vi "P4CMD Dialog - Submit.vi"(6 "changelist files":string[](array[string]), 7 "operation info":T1, 8 "error in (no error)":errorcluster, 9 "description in":string, 10 "input files":string[](array[string])) -> (0 "error out":errorcluster, 1 "description out":string, 2 "filtered file list":string[](array[string]), 5 "dialog box cancelled?":bool)   [LabVIEW 2017, in "NI_SCC_P4CMD.lvlib"]
uses:
  <vilib>/SourceControl/Providers/P4CMD/NI_SCC_P4CMD.lvlib
  <vilib>/SourceControl/support/SCCSup Message Strings GLBL.vi
panel:
  out "submit msg":string="Submit open files to the depot"
  out "Changelist:":string
  out "Date:":string
  out "Client:":string
  out "User:":string
  out "Status:":string
  in  "Description:":string="<enter description here>"
  in  "Cancel":bool
  in  "OK":bool
  in  "Help":bool
  in  "CheckNone":bool
  in  "CheckAll":bool
  in  "Files:":i32[](listbox)
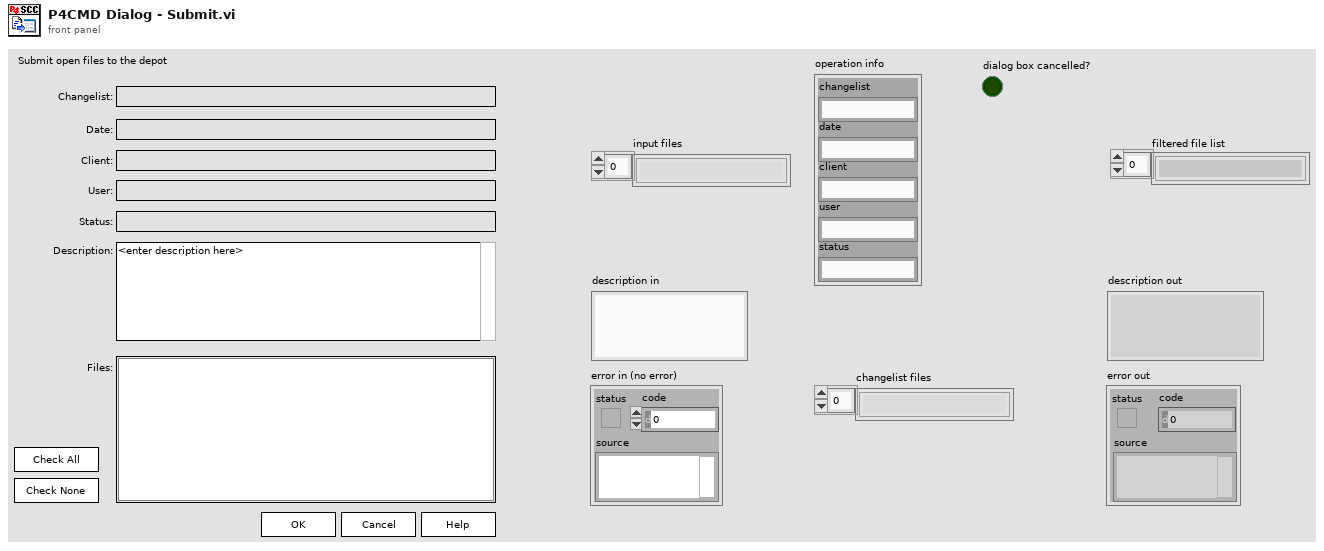
[diagram p1: front panel]
types:
  T1 = cluster{"changelist":string, "date":string, "client":string, "user":string, "status":string}
  T2 = enum16{"Get Checked Symbol", "Get Unchecked Symbol", "Toggle Symbol"}
  T3 = cluster{"Left Button Key Shortcut":cluster{"Control":bool, "Shift":bool, "Key":string}, "Center Button Key Shortcut":cluster{"Control":bool, "Shift":bool, "Key":string}, "Right Button Key Shortcut":cluster{"Control":bool, "Shift":bool, "Key":string}}
  T4 = enum32{"Invalid", "Standard", "Closed", "Hidden", "Minimized", "Maximized"}
  T5 = typedef "LVPoint32TypeDef.ctl" = cluster{"Horizontal":i32, "Vertical":i32}
  T6 = enum16{"Left Button", "Center Button", "Right Button", "Window Close"}
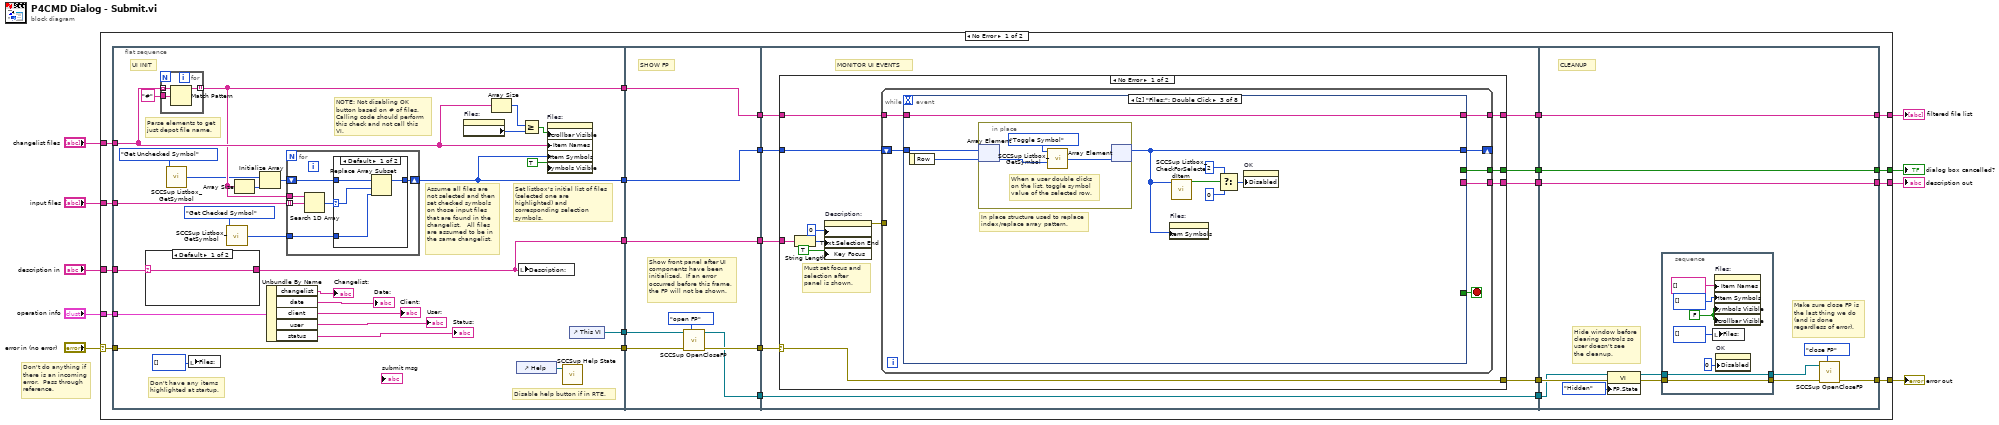
[diagram p0: block diagram]
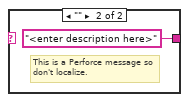
[diagram p2: hidden frame]
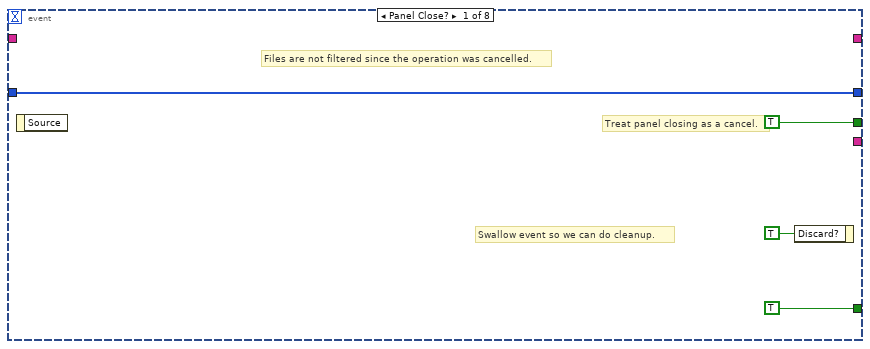
[diagram p4: hidden frame]
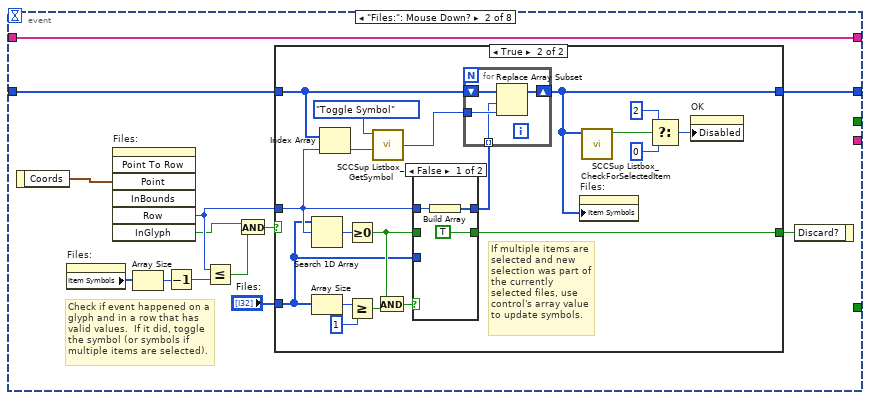
[diagram p5: hidden frame]
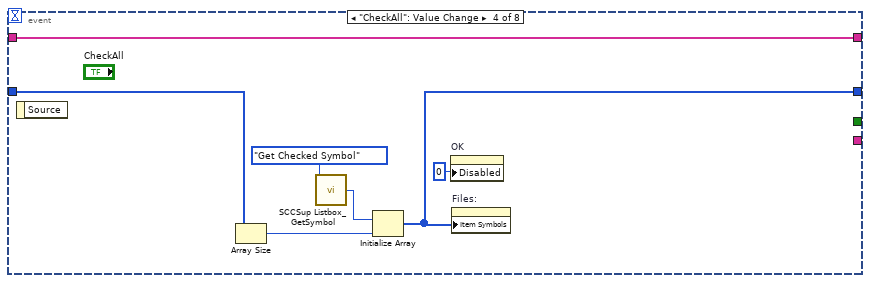
[diagram p8: hidden frame]
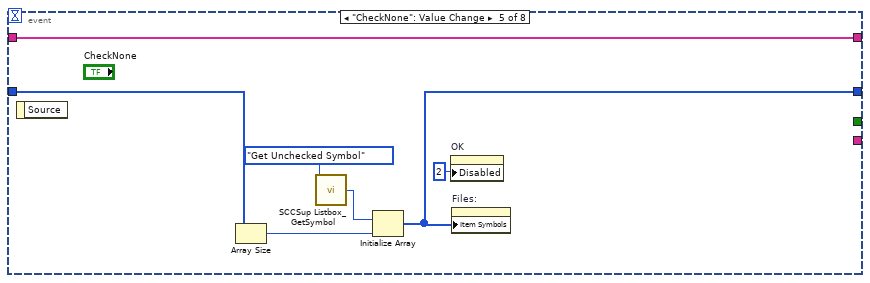
[diagram p9: hidden frame]
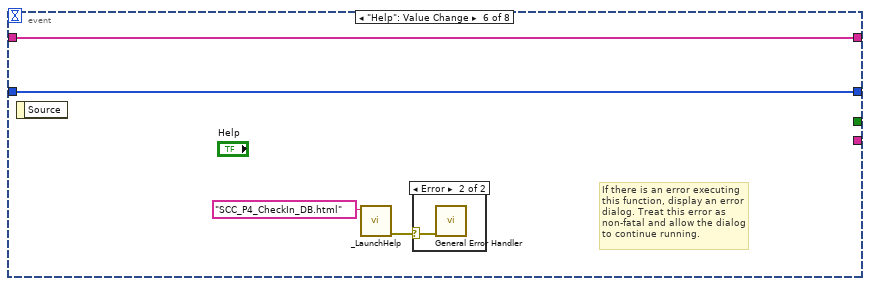
[diagram p10: hidden frame]
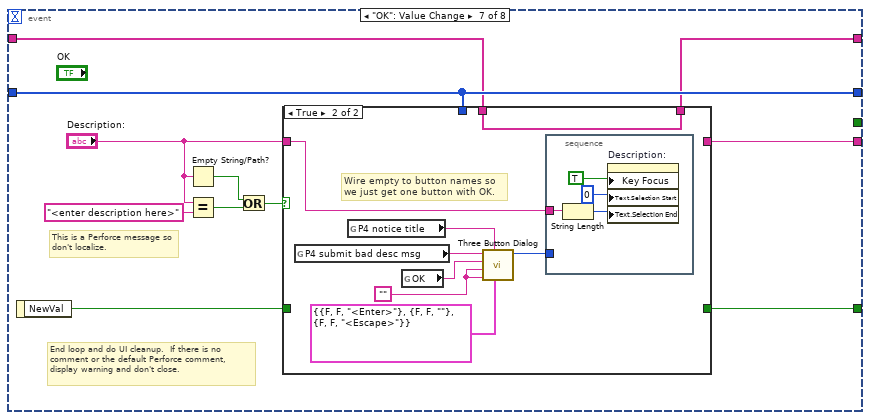
[diagram p12: hidden frame]
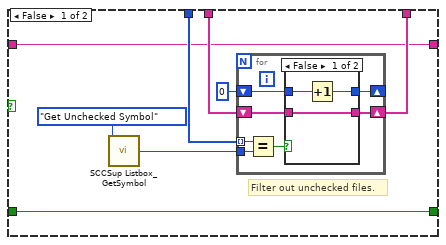
[diagram p13: hidden frame]
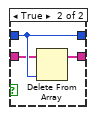
[diagram p14: hidden frame]
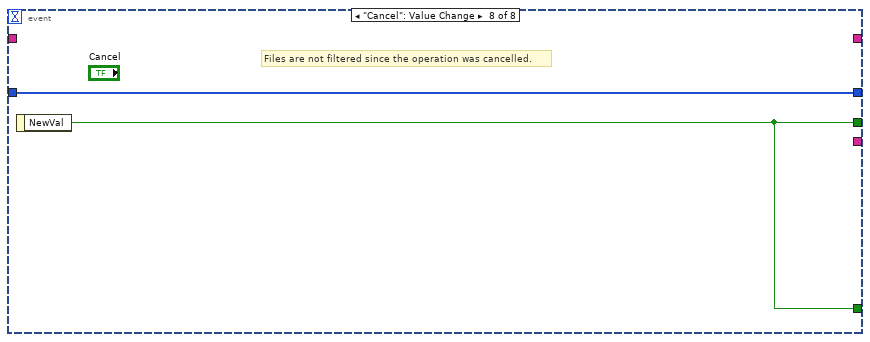
[diagram p15: hidden frame]
diagram:
  # "Don't do anything if there is an incoming error.  Pass through reference."
  n1 = case shown="No Error" "error in (no error)" {
    selector: "error in (no error)" -> [w20 w254]
    tunnel: [w24 w254] -> w9
    tunnel: [w23 _] -> w1
    tunnel: [w22 _] -> w8
    tunnel: [w21 _] -> w7
    tunnel: "input files" -> [w17 _]
    tunnel: "operation info" -> [w16 _]
    tunnel: "description in" -> [w15 _]
    tunnel: "changelist files" -> [w14 _]
    frame No Error {
      n2 = flat-sequence {
        tunnel: [w38] -> w33
        tunnel: [w40] -> w32
        tunnel: [w37] -> w31
        tunnel: w20 -> [w38]
        tunnel: [w47] -> w19
        tunnel: w17 -> [w46]
        tunnel: w16 -> [w57]
        tunnel: w15 -> [w39]
        tunnel: w14 -> [w51]
        tunnel: [w34] -> w11
        tunnel: w33 -> [w82]
        tunnel: w32 -> [w84]
        tunnel: [w84] -> w30
        tunnel: [w83] -> w29
        tunnel: w31 -> [w81]
        tunnel: w19 -> [w83]
        tunnel: [w79] -> w18
        tunnel: [w78] -> w13
        tunnel: w11 -> [w77]
        tunnel: [w77] -> w10
        tunnel: w30 -> [w92]
        tunnel: w29 -> [w93]
        tunnel: [w87] -> w28
        tunnel: [w91] -> w27
        tunnel: [w90] -> w26
        tunnel: [w89] -> w25
        tunnel: w18 -> [w88]
        tunnel: w13 -> [w86]
        tunnel: [w86] -> w12
        tunnel: w10 -> [w85]
        tunnel: [w235] -> w24
        tunnel: w28 -> [w246]
        tunnel: [w244] -> w23
        tunnel: w27 -> [w244]
        tunnel: w26 -> [w243]
        tunnel: [w243] -> w22
        tunnel: w25 -> [w242]
        tunnel: [w242] -> w21
        tunnel: w12 -> [w240]
        frame #0 {
          # "Disable help button if in RTE."
          # "Set listbox's initial list of files (selected one are highlighted) and corresponding selection symbols."
          # "Assume all files are not selected and then set checked symbols on those input files that are found in the changelist.   All files are assumed to be in the same changelist."
          # "Don't have any items highlighted at startup."
          # "Parse elements to get just depot file name."
          # "UI INIT"
          # "NOTE: Not disabling OK button based on # of files.  Calling code should perform this check and not call this VI."
          n3 = case shown="Default" w39 {
            selector: w39 -> [w61 _]
            tunnel: [w61 "<enter description here>" ("Description:")] -> w34
            frame Default {
            }
            frame "" {
              # "This is a Perforce message so don't localize."
            }
          }
          n4 = for {
            tunnel: w51 -> [w76] mode=indexing
            tunnel: [w75] -> w47 mode=indexing
            tunnel: "#" ("regular expression") -> [w74]
            n5 = Match Pattern(string=w76, regular expression=w74) -> (before substring=w75:string)  [unwired: 1 in, 3 out]
          }
          n6 = call <vilib>:"SCCSup Listbox_GetSymbol.vi"("operation"=T2."Get Unchecked Symbol") -> ("symbol out"=w41:i32)  [unwired: 6 in]
          n7 = local write "Files:"(i32[] []) -> ()
          n8 = call <vilib>:"SCCSup Listbox_GetSymbol.vi"("operation"=T2."Get Checked Symbol") -> ("symbol out"=w42:i32)  [unwired: 6 in]
          n9 = Array Size(array=w47) -> (size(s)=w48:i32)
          n10 = Initialize Array(w41, w48) -> (w49:i32[])
          n11 = Unbundle By Name(w57) -> ("changelist"=→"Changelist:":string, "date"=→"Date:":string, "client"=→"Client:":string, "user"=→"User:":string, "status"=→"Status:":string)
          n12 = for {
            tunnel: w47 -> [w68]
            tunnel: w46 -> [w67] mode=indexing
            shift-right: [w64] -> w40
            shift-left: w49 -> [w65]
            tunnel: w42 -> [w63]
            n13 = Search 1D Array(1D array=w68, element=w67) -> (index of element=w66:i32)  [unwired: 1 in]
            n14 = case shown="Default" w66 {
              selector: w66 -> [w70 _]
              tunnel: w65 -> [w72 w73]
              tunnel: [w71 w73] -> w64
              tunnel: w63 -> [w69 _]
              frame Default {
                n15 = Replace Array Subset(array=w72, new element=w69, index=w70) -> (w71:i32[])
              }
              frame -1 {
              }
            }
          }
          n16 = property on="Files:" class="LstBox (strict)"() -> ("Number of Rows"=w36:u32)  [unwired: 2 in, 2 out]
          n17 = Array Size(array=w51) -> (size(s)=w60:i32)
          n18 = control-ref of="Help"() -> (w35:refnum<vi>)
          n19 = local write "Description:"(w34) -> ()
          n20 = Greater Or Equal?(x=w60, y=w36) -> (x >= y?=w58:bool)
          n21 = property on="Files:" class="LstBox (strict)"("Scrollbar Visible"=w58, "Item Names"=w51, "Item Symbols"=w40, "Symbols Visible"=TRUE) -> ()  [unwired: 2 in, 2 out]
          n22 = call <vilib>:"SCCSup Help State.vi"("help ref"=w35) -> ()  [unwired: 10 in, 1 out]
          n23 = control-ref of="This VI"() -> (w37:refnum<vi>)
        }
        frame #1 {
          # "SHOW FP"
          # "Show front panel after UI components have been initialized.  If an error occurred before this frame, the FP will not be shown."
          n24 = call <vilib>:"SCCSup OpenCloseFP.vi"("function"=enum16{"open FP", "close FP"}."open FP", "error in (no error)"=w82, "VI Refnum in"=w81) -> ("error out"=w79:errorcluster, "VI Refnum out"=w78:refnum<vi>)  [unwired: 7 in]
        }
        frame #2 {
          # "MONITOR UI EVENTS"
          n25 = case shown="No Error" w88 {
            selector: w88 -> [w99 w234]
            tunnel: w93 -> [w104 _]
            tunnel: w92 -> [w103 _]
            tunnel: [w102 _] -> w91
            tunnel: [w101 _] -> w90
            tunnel: [w100 _] -> w89
            tunnel: [w99 w234] -> w87
            tunnel: w85 -> [w95 _]
            frame No Error {
              # "Must set focus and selection after panel is shown."
              n26 = String Length(string=w95) -> (length=w98:i32)
              n27 = property on="Description:" class="Str"("Text.Selection Start"=u32 0 ("Text.Selection:Start"), "Text.Selection End"=w98, "Key Focus"=TRUE) -> (error out=w94:errorcluster)  [unwired: 2 in, 1 out]
              n28 = while {
                tunnel: w104 -> [w111]
                shift-right: [w109] -> _
                shift-left: w103 -> [w110]
                tunnel: [w108] -> w102
                tunnel: [w107] -> w101
                tunnel: [w105] -> w100
                tunnel: w94 -> [_]
                stop <- w106 stop-if-true
                n29 = event shown="[2] \"Files:\": Double Click" {
                  selector: _ -> [_ _ _ _ _ _ _ _]
                  dyn-events: _ -> [_ _ _ _ _ _ _ _]
                  timeout: _ -> [_ _ _ _ _ _ _ _]
                  tunnel: w111 -> [_ w125 w165 w175 w182 w186 w197 _]
                  tunnel: w110 -> [w115 w119 w160 w172 w177 w185 w198 w232]
                  tunnel: [w115 w121 w158 w169 w176 w185 w198 w232] -> w109
                  tunnel: [_ w125 w165 w175 w182 w186 w196 _] -> w108
                  tunnel: [TRUE ("Discard?") _ _ _ _ _ _ w233] -> w107
                  tunnel: [TRUE ("Discard?") _ _ _ _ _ w188 w233] -> w106
                  tunnel: [_ _ _ _ _ _ w193 _] -> w105
                  event Panel Close? {
                    # "Treat panel closing as a cancel."
                    # "Files are not filtered since the operation was cancelled."
                    # "Swallow event so we can do cleanup."
                    n30 = event-data() -> ()  [unwired: 1 in, 1 out]
                    n31 = event-data("Discard?"=TRUE) -> ()  [unwired: 1 in, 1 out]
                  }
                  event "Files:": Mouse Down? {
                    # "Check if event happened on a glyph and in a row that has valid values.  If it did, toggle the symbol (or symbols if multiple items are selected)."
                    n32 = event-data() -> ("Coords"=w116:T5)  [unwired: 1 in]
                    n33 = property on="Files:" class="LstBox (strict)"() -> ("Item Symbols"=w128:i32[])  [unwired: 2 in, 2 out]
                    n34 = invoke on="Files:" class="LstBox (strict)" method="Point To Row"("Point"=w116) -> ("Row"=w118:i32, "InGlyph"=w117:bool)  [unwired: 6 in, 5 out]
                    n35 = Array Size(array=w128) -> (size(s)=w120:i32)
                    n36 = Decrement(x=w120) -> (x-1=w127:i32)
                    n37 = Less Or Equal?(x=w118, y=w127) -> (x <= y?=w126:bool)
                    n38 = And(x=w117, y=w126) -> (x .and. y?=w124:bool)
                    n39 = case shown="True" w124 {
                      tunnel: "Files:" -> [_ w139]
                      tunnel: w118 -> [_ w140]
                      tunnel: w119 -> [w129 w137]
                      tunnel: [_ w138] -> w122
                      tunnel: [w129 w134] -> w121
                      frame False {
                      }
                      frame True {
                        # "If multiple items are selected and new selection was part of the currently selected files, use control's array value to update symbols."
                        n40 = Search 1D Array(1D array=w139, element=w140) -> (index of element=w146:i32)  [unwired: 1 in]
                        n41 = Array Size(array=w139) -> (size(s)=w148:i32)
                        n42 = Index Array(array=w137, index=w140) -> (element=w144:i32)
                        n43 = Greater Or Equal To 0?(x=w146) -> (x >= 0?=w141:bool)
                        n44 = Greater Or Equal?(x=w148, y=1) -> (x >= y?=w145:bool)
                        n45 = call <vilib>:"SCCSup Listbox_GetSymbol.vi"("operation"=T2."Toggle Symbol", "symbol in"=w144) -> ("symbol out"=w136:i32)  [unwired: 5 in]
                        n46 = And(x=w141, y=w145) -> (x .and. y?=w142:bool)
                        n47 = case shown="False" w142 {
                          tunnel: w141 -> [_ w156]
                          tunnel: w140 -> [w155 _]
                          tunnel: w139 -> [_ w157]
                          tunnel: [w154 w157] -> w135
                          tunnel: [TRUE w156] -> w138
                          frame False {
                            n48 = Build Array(w155) -> (w154:i32[])
                          }
                          frame True {
                          }
                        }
                        n49 = for {
                          shift-right: [w151] -> w134
                          shift-left: w137 -> [w152]
                          tunnel: w136 -> [w150]
                          tunnel: w135 -> [w149] mode=indexing
                          n50 = Replace Array Subset(array=w152, new element=w150, index=w149) -> (w151:i32[])
                        }
                        n51 = property on="Files:" class="LstBox (strict)"("Item Symbols"=w134) -> ()  [unwired: 2 in, 2 out]
                        n52 = call <vilib>:"SCCSup Listbox_CheckForSelectedItem.vi"("symbols array"=w134) -> ("item selected?"=w131:bool)  [unwired: 9 in, 1 out]
                        n53 = Select(t=u8 2 ("Disabled"), s=w131, f=u8 0) -> (s? t:f=w130:u8)
                        n54 = property on="OK" class="Bool"("Disabled"=w130) -> ()  [unwired: 2 in, 2 out]
                      }
                    }
                    n55 = event-data("Discard?"=w122) -> ()  [unwired: 1 in, 1 out]
                  }
                  event "Files:": Double Click {
                    # "In place structure used to replace index/replace array pattern."
                    n56 = event-data() -> ("Row"=w159:i32)  [unwired: 1 in]
                    n57 = in-place {
                      # "When a user double clicks on the list, toggle symbol value of the selected row."
                      n58 = in-place-array #1(w160, w159) -> (w167:i32)
                      n59 = call <vilib>:"SCCSup Listbox_GetSymbol.vi"("operation"=T2."Toggle Symbol", "symbol in"=w167) -> ("symbol out"=w166:i32)  [unwired: 5 in]
                      n60 = in-place-array #1(w166) -> (w158:i32[])  [unwired: 1 out]
                    }
                    n61 = property on="Files:" class="LstBox (strict)"("Item Symbols"=w158) -> ()  [unwired: 2 in, 2 out]
                    n62 = call <vilib>:"SCCSup Listbox_CheckForSelectedItem.vi"("symbols array"=w158) -> ("item selected?"=w162:bool)  [unwired: 9 in, 1 out]
                    n63 = Select(t=u8 2 ("Disabled"), s=w162, f=u8 0) -> (s? t:f=w161:u8)
                    n64 = property on="OK" class="Bool"("Disabled"=w161) -> ()  [unwired: 2 in, 2 out]
                  }
                  event "CheckAll": Value Change {
                    n65 = event-data() -> ()  [unwired: 1 in, 1 out]
                    n66 = Array Size(array=w172) -> (size(s)=w171:i32)
                    n67 = call <vilib>:"SCCSup Listbox_GetSymbol.vi"("operation"=T2."Get Checked Symbol") -> ("symbol out"=w170:i32)  [unwired: 6 in]
                    n68 = Initialize Array(w170, w171) -> (w169:i32[])
                    n69 = property on="OK" class="Bool"("Disabled"=u8 0) -> ()  [unwired: 2 in, 2 out]
                    n70 = property on="Files:" class="LstBox (strict)"("Item Symbols"=w169) -> ()  [unwired: 2 in, 2 out]
                  }
                  event "CheckNone": Value Change {
                    n71 = event-data() -> ()  [unwired: 1 in, 1 out]
                    n72 = Array Size(array=w177) -> (size(s)=w179:i32)
                    n73 = call <vilib>:"SCCSup Listbox_GetSymbol.vi"("operation"=T2."Get Unchecked Symbol") -> ("symbol out"=w178:i32)  [unwired: 6 in]
                    n74 = Initialize Array(w178, w179) -> (w176:i32[])
                    n75 = property on="OK" class="Bool"("Disabled"=u8 2) -> ()  [unwired: 2 in, 2 out]
                    n76 = property on="Files:" class="LstBox (strict)"("Item Symbols"=w176) -> ()  [unwired: 2 in, 2 out]
                  }
                  event "Help": Value Change {
                    # "If there is an error executing this function, display an error dialog. Treat this error as non-fatal and allow the dialog to continue running."
                    n77 = event-data() -> ()  [unwired: 1 in, 1 out]
                    n78 = call <helpdir>:"_LaunchHelp.vi"("HTML filename"="SCC_P4_CheckIn_DB.html" ("Help topic")) -> ("error out"=w184:errorcluster)  [unwired: 6 in]
                    n79 = case shown="Error" w184 {
                      selector: w184 -> [_ w187]
                      frame No Error {
                      }
                      frame Error {
                        n80 = call <vilib>:"General Error Handler.vi"("error in (no error)"=w187) -> ()  [unwired: 10 in, 5 out]
                      }
                    }
                  }
                  event "OK": Value Change {
                    # "This is a Perforce message so don't localize."
                    # "End loop and do UI cleanup.  If there is no comment or the default Perforce comment, display warning and don't close."
                    n81 = event-data() -> ("NewVal"=w189:bool)  [unwired: 1 in]
                    n82 = Empty String/Path?(string/path="Description:") -> (empty?=w191:bool)
                    n83 = Equal?(x="Description:", y="<enter description here>" ("Description:")) -> (x = y?=w190:bool)
                    n84 = Or(x=w191, y=w190) -> (x .or. y?=w195:bool)
                    n85 = case shown="True" w195 {
                      tunnel: w198 -> [w203 _]
                      tunnel: w197 -> [w202 w227]
                      tunnel: [w201 w227] -> w196
                      tunnel: "Description:" -> [w200 w226]
                      tunnel: [w200 _] -> w193
                      tunnel: w189 -> [w199 _]
                      tunnel: [w199 _] -> w188
                      frame False {
                        # "Filter out unchecked files."
                        n86 = call <vilib>:"SCCSup Listbox_GetSymbol.vi"("operation"=T2."Get Unchecked Symbol") -> ("symbol out"=w206:i32)  [unwired: 6 in]
                        n87 = for {
                          tunnel: w206 -> [w213]
                          tunnel: w203 -> [w212] mode=indexing
                          shift-right: [w209] -> w201
                          shift-left: w202 -> [w210]
                          shift-right: [w207] -> _
                          shift-left: 0 -> [w208]
                          n88 = Equal?(x=w212, y=w213) -> (x = y?=w211:bool)
                          n89 = case shown="False" w211 {
                            tunnel: w210 -> [w216 w217]
                            tunnel: [w216 w219] -> w209
                            tunnel: w208 -> [w215 w218]
                            tunnel: [w214 w218] -> w207
                            frame False {
                              n90 = Increment(x=w215) -> (x+1=w214:i32)
                            }
                            frame True {
                              n91 = Delete From Array(array=w217, index=w218) -> (array with subset deleted=w219:string[])  [unwired: 1 in, 1 out]
                            }
                          }
                        }
                      }
                      frame True {
                        w222 = ""
                        # "Wire empty to button names so we just get one button with OK."
                        n92 = global read "SCCSup Message Strings GLBL.vi" "P4 submit bad desc msg"() -> (w224:string)
                        n93 = global read "SCCSup Message Strings GLBL.vi" "P4 notice title"() -> (w225:string)
                        n94 = global read "SCCSup Message Strings GLBL.vi" "OK"() -> (w221:string)
                        n95 = call <vilib>:"Three Button Dialog.vi"("Keyboard Shortcuts (Left is <Enter>)"=T3 {"Left Button Key Shortcut"={"Control"=FALSE, "Shift"=FALSE, "Key"="<Enter>"}, "Center Button Key Shortcut"={"Control"=FALSE, "Shift"=FALSE, "Key"=""}, "Right Button Key Shortcut"={"Control"=FALSE, "Shift"=FALSE, "Key"="<Escape>"}}, "Window Title (\"\")"=w225, "Right Button Text (\"Cancel\")"=w222, "Center Button Text (\"No\")"=w222, "Left Button Text (\"Yes\")"=w221, "message"=w224) -> ("Which Button?"=w223:T6)  [unwired: 5 in]
                        n96 = stacked-sequence {
                          tunnel: w226 -> [w229]
                          tunnel: w223 -> [_]
                          frame #0 {
                            n97 = String Length(string=w229) -> (length=w230:i32)
                            n98 = property on="Description:" class="Str"("Key Focus"=TRUE, "Text.Selection Start"=u32 0 ("Text.Selection:Start"), "Text.Selection End"=w230) -> ()  [unwired: 2 in, 2 out]
                          }
                        }
                      }
                    }
                  }
                  event "Cancel": Value Change {
                    # "Files are not filtered since the operation was cancelled."
                    n99 = event-data() -> ("NewVal"=w233:bool)  [unwired: 1 in]
                  }
                }
              }
            }
            frame Error {
              # "If there was an error upstream, don't run UI monitor code.  Pass error through and let caller handle the error."
            }
          }
        }
        frame #3 {
          # "CLEANUP"
          # "Hide window before clearing controls so user doesn't see the cleanup."
          # "Make sure close FP is the last thing we do (and is done regardless of error)."
          n100 = property class="VI"(reference=w240, error in=w246, "FP.State"=T4."Hidden" ("Front Panel Window:State")) -> (reference out=w239:refnum<vi>, error out=w241:errorcluster)
          n101 = stacked-sequence {
            tunnel: w241 -> [w248]
            tunnel: [w248] -> w236
            tunnel: w239 -> [w247]
            tunnel: [w247] -> w237
            frame #0 {
              w251 = FALSE ("Symbols Visible")
              n102 = local write "Files:"(i32[] [] ("Files:")) -> ()
              n103 = property on="Files:" class="LstBox (strict)"("Item Names"=string[] [], "Item Symbols"=i32[] [], "Symbols Visible"=w251, "Scrollbar Visible"=w251) -> ()  [unwired: 2 in, 2 out]
              n104 = property on="OK" class="Bool"("Disabled"=u8 0) -> ()  [unwired: 2 in, 2 out]
            }
          }
          n105 = call <vilib>:"SCCSup OpenCloseFP.vi"("function"=enum16{"open FP", "close FP"}."close FP", "error in (no error)"=w236, "VI Refnum in"=w237) -> ("error out"=w235:errorcluster)  [unwired: 7 in, 1 out]
        }
      }
    }
    frame Error {
    }
  }
  "error out" <- w9
  "description out" <- w7
  "dialog box cancelled?" <- w8
  "filtered file list" <- w1
